vi "Reset Chips.vi"(8 "error in (no error)":errorcluster, 11 "RT data":T1 {"DIO Engine Refs"."RT IDs"."Slot #" max=15; "DIO Engine Refs"."RT IDs"."Chip Address (A2 A1 A0)" max=7; "DIO Engine Refs"."RT Block Data Refs"."Data Reference" format="%.0x"; "LED Engine Refs"."RT IDs"."Slot #" max=15; "LED Engine Refs"."RT IDs"."Chip Address (A2 A1 A0)" max=7; "LED Engine Refs"."RT Block Data Refs"."Data Reference" format="%.0x"; "Current Sense Engine Refs"."RT IDs"."Slot #" max=15; "Current Sense Engine Refs"."RT IDs"."Chip Address (A2 A1 A0)" max=7; "Current Sense Engine Refs"."RT Block Data Refs"."Data Reference" format="%.0x"; "Resistor Engine Refs"."RT IDs"."Slot #" max=15; "Resistor Engine Refs"."RT IDs"."Chip Address (A2 A1 A0)" max=7; "Resistor Engine Refs"."RT Block Data Refs"."Data Reference" format="%.0x"; "Wheel Speed Sensor Engine Refs"."RT IDs"."Slot #" max=15; "Wheel Speed Sensor Engine Refs"."RT IDs"."Chip Address (A2 A1 A0)" max=7; "Wheel Speed Sensor Engine Refs"."RT Block Data Refs"."Data Reference" format="%.0x"; "Battery Switch Engine Refs"."RT IDs"."Slot #" max=15; "Battery Switch Engine Refs"."RT IDs"."Chip Address (A2 A1 A0)" max=7; "Battery Switch Engine Refs"."RT Block Data Refs"."Data Reference" format="%.0x"; "FIU Engine Refs"."RT IDs"."Slot #" max=15; "FIU Engine Refs"."RT IDs"."Chip Address (A2 A1 A0)" max=7; "FIU Engine Refs"."RT Block Data Refs"."Data Reference" format="%.0x"}) -> (0 "error out":errorcluster)   [LabVIEW 2014, in "SLSC configuration Shared.lvlib"]
uses:
  SLSC configuration Shared.lvlib
  Engine/Type Defs/RT data.ctl
  Engine/Type Defs/RT Engine Refs.ctl
  Type Defs/RT IDs.ctl
  Slot #.ctl
  MCP23S17/Chip Address.ctl
  <vilib>/NI Veristand/Custom Device API/Block Data Reference.ctl
  <vilib>/NI Veristand/Custom Device API/Data Reference.ctl
  Engine/SLSC configuration Engine.lvlib
  <vilib>/NI Veristand/Custom Device API/Custom Device API.lvlib
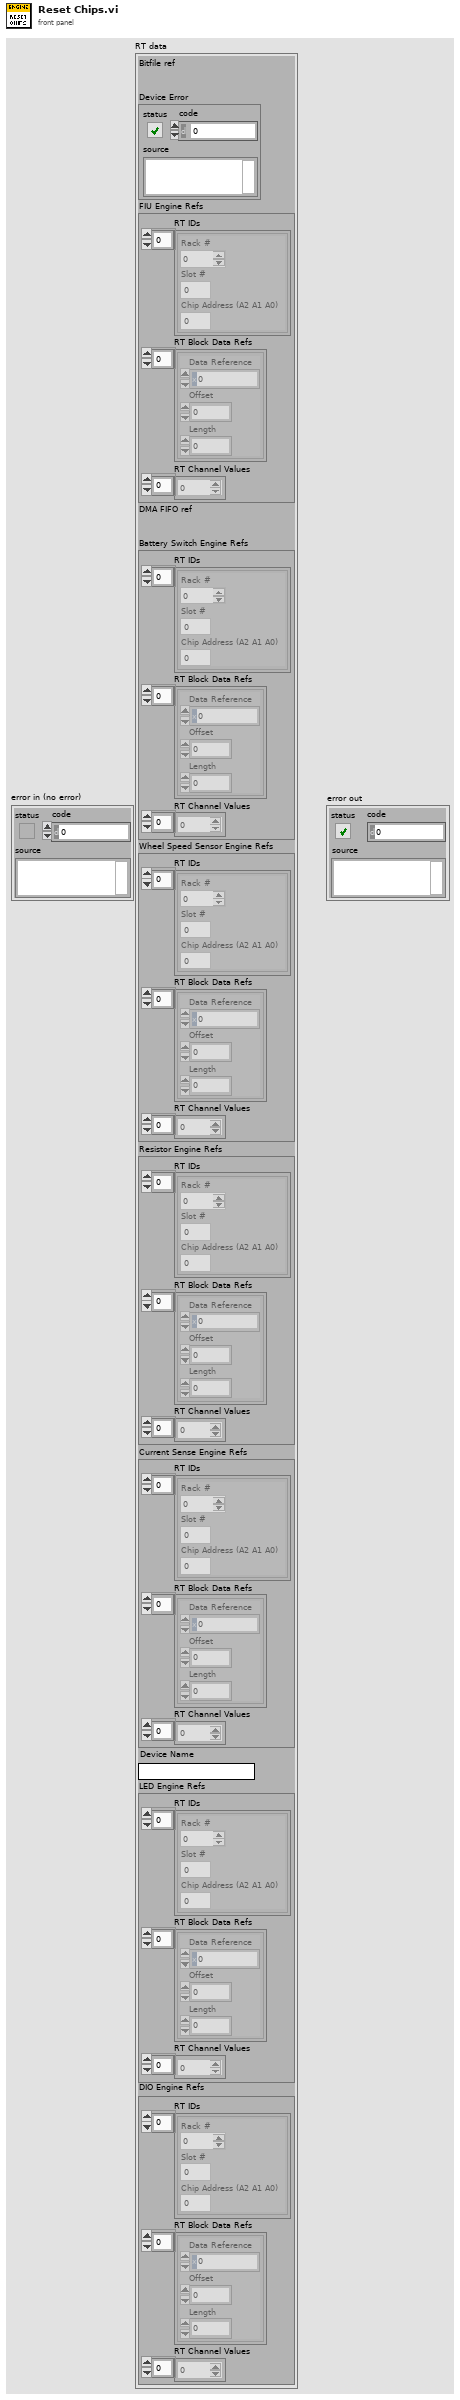
[diagram p1: front panel]
types:
  T1 = typedef "SLSC configuration Engine.lvlib/RT data.ctl" = cluster{"Bitfile ref":refnum<k20>, "Device Error":errorcluster, "FIU Engine Refs":T2, "DMA FIFO ref":refnum<k20>, "Battery Switch Engine Refs":T2, "Wheel Speed Sensor Engine Refs":T2, "Resistor Engine Refs":T2, "Current Sense Engine Refs":T2, "Device Name":string, "LED Engine Refs":T2, "DIO Engine Refs":T2}
  T2 = typedef "SLSC configuration Engine.lvlib/RT Engine Refs.ctl" = cluster{"RT IDs":T3[], "RT Block Data Refs":T6[], "RT Channel Values":dbl[]}
  T3 = typedef "SLSC configuration Shared.lvlib/RT IDs.ctl" = cluster{"Rack #":u8, "Slot #":T4, "Chip Address (A2 A1 A0)":T5}
  T4 = typedef "SLSC configuration Shared.lvlib/Slot #.ctl" = u8
  T5 = typedef "SLSC configuration Shared.lvlib/Chip Address.ctl" = u8
  T6 = typedef "Custom Device API.lvlib/Block Data Reference.ctl" = cluster{"Data Reference":T7, "Offset":i32, "Length":i32}
  T7 = typedef "Custom Device API.lvlib/Data Reference.ctl" = i32
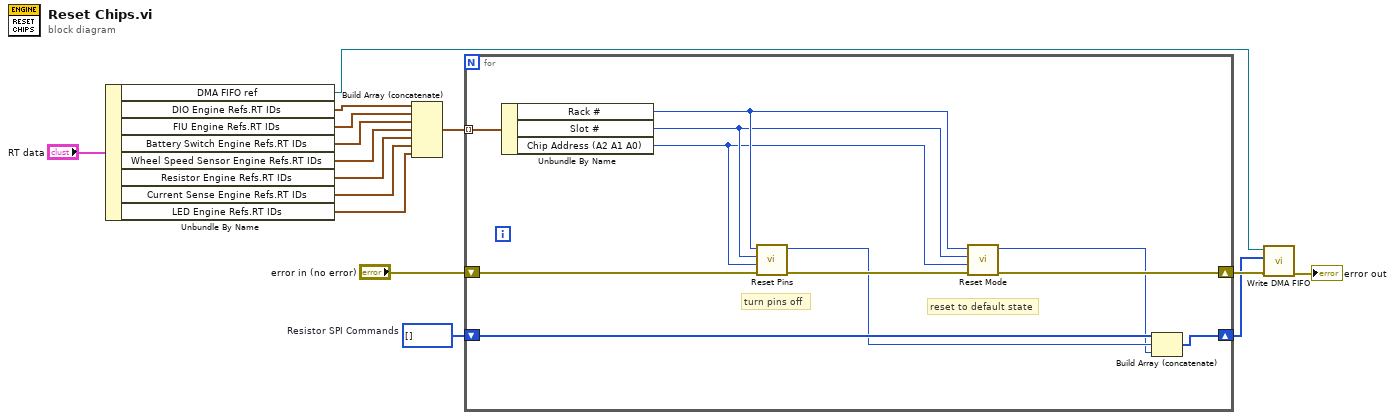
[diagram p0: block diagram]
diagram:
  w15 = u64[] []  # Resistor SPI Commands
  n1 = Unbundle By Name("RT data") -> ("DMA FIFO ref"=w2:refnum<k20>, "DIO Engine Refs.RT IDs"=w1:T3[], "FIU Engine Refs.RT IDs"=w9:T3[], "Battery Switch Engine Refs.RT IDs"=w8:T3[], "Wheel Speed Sensor Engine Refs.RT IDs"=w7:T3[], "Resistor Engine Refs.RT IDs"=w6:T3[], "Current Sense Engine Refs.RT IDs"=w5:T3[], "LED Engine Refs.RT IDs"=w4:T3[])
  n2 = Build Array (concatenate)(w1, w9, w8, w7, w6, w5, w4) -> (w3:T3[])
  n3 = for {
    shift-right: [w19] -> w14
    shift-left: "error in (no error)" -> [w24]
    tunnel: w3 -> [w26] mode=indexing
    shift-right: [w16] -> w13
    shift-left: w15 -> [w25]
    # "reset to default state"
    # "turn pins off"
    n4 = Unbundle By Name(w26) -> ("Rack #"=w22:u8, "Slot #"=w21:T4, "Chip Address (A2 A1 A0)"=w20:T5)
    n5 = call "Reset Pins.vi"("error in (no error)"=w24, "Chip Address (A2 A1 A0)"=w20, "Slot #"=w21, "Rack #"=w22) -> ("error out"=w23:errorcluster, "SPI FIFO Message"=w18:u64)  [unwired: 6 in]
    n6 = call "Reset Mode.vi"("error in (no error)"=w23, "Chip Address (A2 A1 A0)"=w20, "Slot #"=w21, "Rack #"=w22) -> ("error out"=w19:errorcluster, "SPI FIFO Message"=w17:u64)  [unwired: 6 in]
    n7 = Build Array (concatenate)(w25, w18, w17) -> (w16:u64[])
  }
  n8 = call "Write DMA FIFO.vi"("error in (no error)"=w14, "FIU SPI Commands"=w13, "DMA FIFO Ref in"=w2) -> ("error out"=→"error out":errorcluster)  [unwired: 8 in]
